vi "DoubleSolenoid_Pulse_Execute.vi"(4 "Pass_Through_Time":dbl=-1.0 format="%33.4f", 6 "Solenoid Pulse\nTime Seconds":dbl=1.5 format="%#_13g", 9 "Solenoid Demand":bool, 11 "Robot Enabled":bool) -> (3 "Solenoid Cmd":T1)   [LabVIEW 2019, in "Trajectory_Library.lvlib"]
uses:
  Trajectory_Library.lvlib
  <vilib>/Rock Robotics/WPI/Solenoid/WPI_SolenoidValue.ctl
  Util_GetTime_U32.vi
  Timer_New.vi
  Util_GetTime_U64.vi
  <vilib>/Utility/semaphor.llb/Obtain Semaphore Reference.vi
  Timer_Reset.vi
  Timer_Start.vi
  Timer_HasPeriodPassedOnce.vi
  Timer_Stop.vi
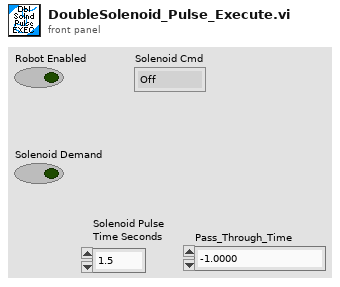
[diagram p1: front panel]
types:
  T1 = typedef "WPI_SolenoidValue.ctl" = enum16{"Off", "On", "Forward", "Reverse"}
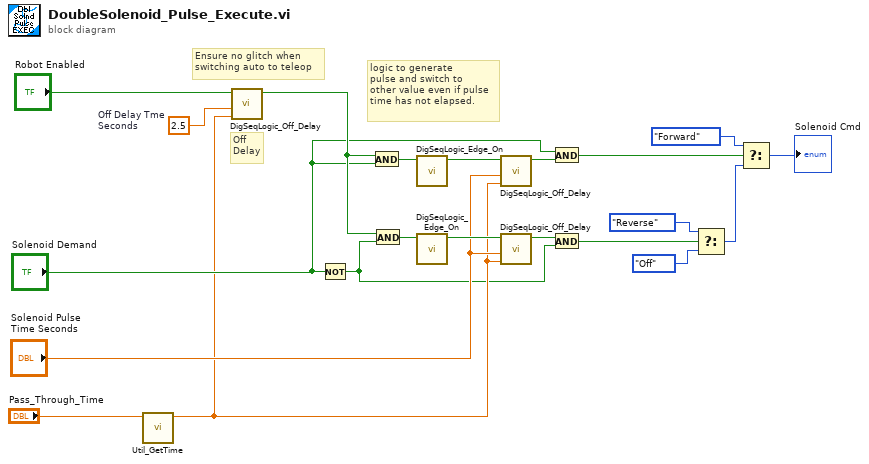
[diagram p0: block diagram]
diagram:
  w15 = 2.5  # Off Delay Tme Seconds
  # "logic to generate \npulse and switch to\nother value even if pulse\ntime has not elapsed."
  # "Ensure no glitch when\nswitching auto to teleop"
  # "Off \nDelay"
  n1 = call "Util_GetTime.vi"("Pass_Through_Time"="Pass_Through_Time") -> ("FPGA_Time_Seconds"=w5:dbl)  [unwired: 8 in, 2 out]
  n2 = call "DigSeqLogic_Off_Delay.vi"("Time"=w5, "Delay"=w15, "Input"="Robot Enabled") -> ("Output"=w16:bool)  [unwired: 7 in, 1 out]
  n3 = Not(x="Solenoid Demand") -> (.not. x?=w3:bool)
  n4 = And(x=w16, y="Solenoid Demand") -> (x .and. y?=w12:bool)
  n5 = And(x=w16, y=w3) -> (x .and. y?=w7:bool)
  n6 = call "DigSeqLogic_Edge_On.vi"("Input"=w12) -> ("On Edge"=w11:bool)  [unwired: 10 in]
  n7 = call "DigSeqLogic_Edge_On.vi"("Input"=w7) -> ("On Edge"=w8:bool)  [unwired: 10 in]
  n8 = call "DigSeqLogic_Off_Delay.vi"("Time"=w5, "Delay"="Solenoid Pulse\nTime Seconds", "Input"=w11) -> ("Output"=w10:bool)  [unwired: 7 in, 1 out]
  n9 = call "DigSeqLogic_Off_Delay.vi"("Time"=w5, "Delay"="Solenoid Pulse\nTime Seconds", "Input"=w8) -> ("Output"=w4:bool)  [unwired: 7 in, 1 out]
  n10 = And(x="Solenoid Demand", y=w10) -> (x .and. y?=w1:bool)
  n11 = And(x=w4, y=w3) -> (x .and. y?=w2:bool)
  n12 = Select(t=WPI_SolenoidValue."Reverse" ("Value"), s=w2, f=WPI_SolenoidValue."Off" ("Value")) -> (s? t:f=w19:T1)
  n13 = Select(t=WPI_SolenoidValue."Forward" ("Value"), s=w1, f=w19) -> (s? t:f=→"Solenoid Cmd":T1)
